vi "LoadDIOSettings.vi"(8 "Error in":errorcluster, 10 "Current ExpState IN":T1 {"RIO Settings"."Card Settings"."Sample Rate" format="%#_3p"; "Timing Settings"."Timing Channel Settings"."FrontPanelTime" format="%.3p"; "Timing Settings"."Timing Channel Settings"."Pulse width (s)" format="%.3p"; "Timing Settings"."Timing Channel Settings"."Delay (s)" format="%.3p"; "DAQ Settings"."Card Settings"."Global Edge Type" items=["Rising"=10280, "Falling"=10171]; "DAQ Settings"."Card Settings"."Sample Rate" format="%#_3p"}, 11 "Tree DVR in":refnum<data-value>) -> (0 "Error out":errorcluster, 3 "DIO Settings":T16)   [LabVIEW 2014]
uses:
  Controls/DIOSettingsExperimentStateCluster.ctl
  Controls/DIOChannel.ctl
  <vilib>/MDSplus/Classes/Tree_Class/Tree.lvclass
  Controls/ExperimentStateCluster.ctl
  Controls/DigitizerSettingsChannelSettings.ctl
  Controls/DigitizerSettingsCardSettingsArray.ctl
  Controls/DigitizerSettingsCardSettings.ctl
  Controls/TimingSettings.ctl
  Controls/TimingCardSettings.ctl
  Controls/TimingChannelSettings.ctl
  Controls/RIOSettingsExperimentStateCluster.ctl
  Controls/RIOChannelSettingsArrayExperimentStateCluster.ctl
  Controls/RIOSettingsChannelSettings.ctl
  Controls/RIOSettingsCardSettingsArray.ctl
  Controls/RIOSettingsCardSettings.ctl
  <vilib>/userdefined/High Color/nirio_resource_hc.ctl
  Controls/RIOData.ctl
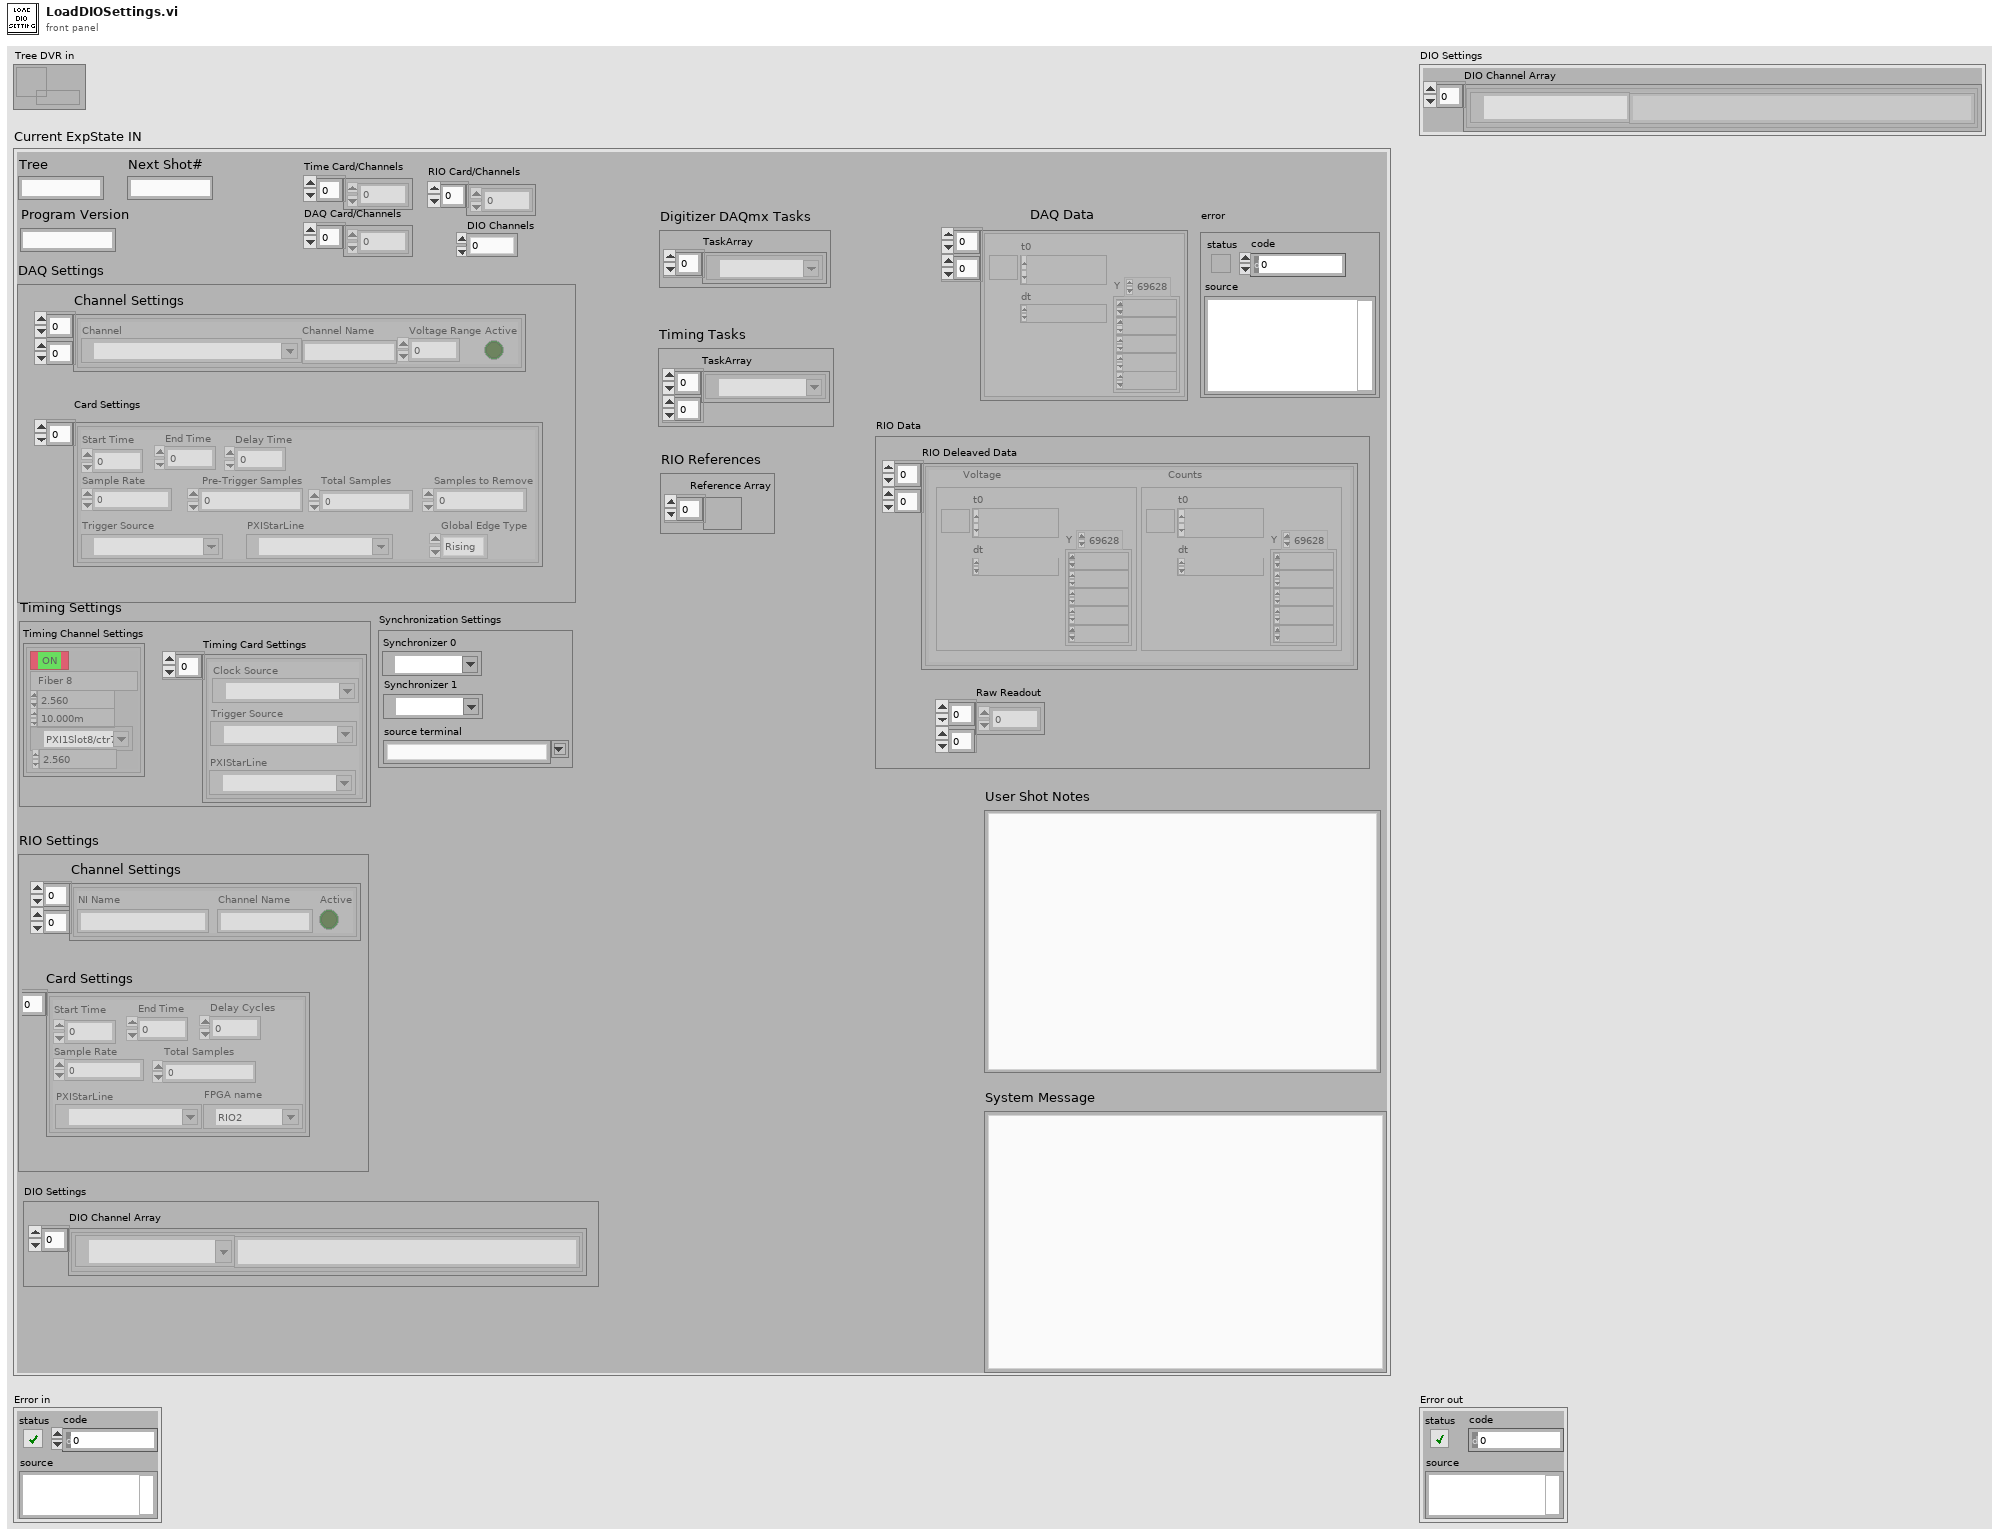
[diagram p1: front panel]
types:
  T1 = typedef "ExperimentStateCluster.ctl" = cluster{"error":errorcluster, "Digitizer DAQmx Tasks":cluster{"TaskArray":refnum<k21>[]}, "DAQ Settings":cluster{"Channel Settings":T2[][], "Card Settings":T3}, "Synchronization Settings":cluster{"Synchronizer 0":refnum<k15>, "source terminal":string, "Synchronizer 1":refnum<k15>}, "DAQ Data":waveform(dbl)[][], "Next Shot#":string, "System Message":string, "User Shot Notes":string, "Timing Settings":T5, "Timing Tasks":cluster{"TaskArray":refnum<k21>[][]}, "Tree":string, "Time Card/Channels":i32[], "DAQ Card/Channels":i32[], "Program Version":string, "RIO Settings":T8, "RIO References":cluster{"Reference Array":refnum<k20>[]}, "RIO Data":T14, "RIO Card/Channels":i32[], "DIO Channels":i32, "DIO Settings":cluster{"DIO Channel Array":T15[]}}
  T2 = typedef "DigitizerSettingsChannelSettings.ctl" = cluster{"Channel":tag, "Channel Name":string, "Voltage Range":dbl, "Active":bool}
  T3 = typedef "DigitizerSettingsCardSettingsArray.ctl" = T4[]
  T4 = typedef "DigitizerSettingsCardSettings.ctl" = cluster{"Start Time":dbl, "End Time":dbl, "Sample Rate":dbl, " Pre-Trigger Samples":u32, "Total Samples":i32, "Samples to Remove":u32, "Trigger Source":tag, "Global Edge Type":i32, "PXIStarLine":tag, "Delay Time":dbl}
  T5 = typedef "TimingSettings.ctl" = cluster{"Timing Card Settings":T6[], "Timing Channel Settings":T7[][]}
  T6 = typedef "TimingCardSettings.ctl" = cluster{"Trigger Source":tag, "Clock Source":tag, "PXIStarLine":tag}
  T7 = typedef "TimingChannelSettings.ctl" = cluster{"Delay (s)":dbl, "Pulse width (s)":dbl, "Active":bool, "Channel Name":string, "counter":tag, "FrontPanelTime":dbl}
  T8 = typedef "RIOSettingsExperimentStateCluster.ctl" = cluster{"Channel Settings":T9, "Card Settings":T11}
  T9 = typedef "RIOChannelSettingsArrayExperimentStateCluster.ctl" = T10[][]
  T10 = typedef "RIOSettingsChannelSettings.ctl" = cluster{"Channel Name":string, "Active":bool, "NI Name":string}
  T11 = typedef "RIOSettingsCardSettingsArray.ctl" = T12[]
  T12 = typedef "RIOSettingsCardSettings.ctl" = cluster{"Start Time":dbl, "End Time":dbl, "Sample Rate":dbl, "Total Samples":u64, "PXIStarLine":tag, "Delay Cycles":u64, "FPGA name":T13}
  T13 = typedef "nirio_resource_hc.ctl" = tag
  T14 = typedef "RIOData.ctl" = cluster{"RIO Deleaved Data":cluster{"Voltage":waveform(dbl), "Counts":waveform(i16)}[][], "Raw Readout":u64[][]}
  T15 = typedef "DIOChannel.ctl" = cluster{"Channel Name":string, "NI Name":tag}
  T16 = typedef "DIOSettingsExperimentStateCluster.ctl" = cluster{"DIO Channel Array":T15[]}
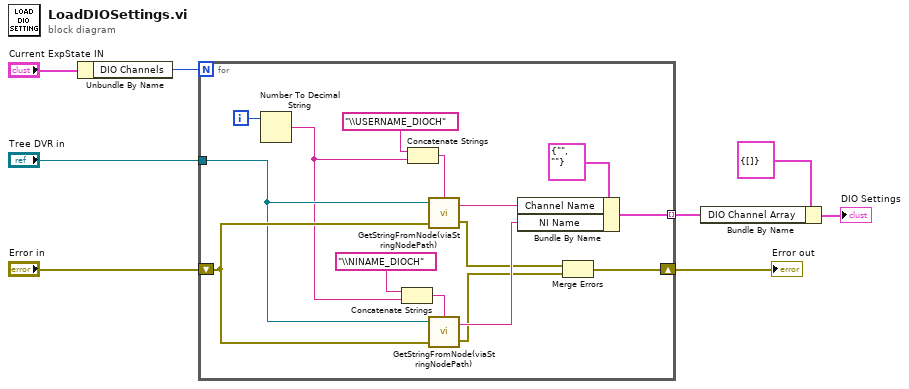
[diagram p0: block diagram]
diagram:
  n1 = Unbundle By Name("Current ExpState IN") -> ("DIO Channels"=w4:i32)
  n2 = for {
    N: w4 -> [_]
    tunnel: "Tree DVR in" -> [w16]
    shift-right: [w22] -> w7
    shift-left: "Error in" -> [w17]
    tunnel: [w23] -> w2 mode=indexing
    i -> [w19]
    n3 = Number To Decimal String(number=w19) -> (decimal integer string=w13:string)  [unwired: 1 in]
    n4 = Concatenate Strings("\\NINAME_DIOCH" ("string"), w13) -> (w12:string)
    n5 = Concatenate Strings("\\USERNAME_DIOCH" ("string"), w13) -> (w15:string)
    n6 = call "GetStringFromNode(viaStringNodePath).vi"("Path"=w15, "error in"=w17, "Tree DVR in"=w16) -> ("error out"=w11:errorcluster, "String out"=w20:string)  [unwired: 1 in]
    n7 = call "GetStringFromNode(viaStringNodePath).vi"("Path"=w12, "error in"=w17, "Tree DVR in"=w16) -> ("error out"=w10:errorcluster, "String out"=w21:string)  [unwired: 1 in]
    n8 = Bundle By Name(cluster=T15 {"Channel Name"="", "NI Name"=""} ("DIO Channels"), "Channel Name"=w20, "NI Name"=w21) -> (w23:T15)
    n9 = Merge Errors(w11, w10) -> (w22:errorcluster)
  }
  "Error out" <- w7
  n10 = Bundle By Name(cluster=T16 {"DIO Channel Array"=[]} ("DIO Settings"), "DIO Channel Array"=w2) -> (→"DIO Settings":T16)
